vi "Get Signal Names.vi"(8 "error in (no error)":errorcluster, 11 "Incoming/Outgoing in":T1 format="%.0x") -> (0 "error out":errorcluster, 1 "signal names":string[](array[string]), 2 "signals":T1[](array[typedef]) format="%.0x", 3 "Incoming/Outgoing out":T1 format="%.0x")   [LabVIEW 2020, in "Communication Bus Template Engine.lvlib" / "Implementation.lvlib" / "Execution Unit Factory.lvclass"]
uses:
  Execution Unit Factory.lvclass
  Scripting/Communication Bus Template Scripting.lvlib
  <vilib>/NI VeriStand/Custom Device API/Custom Device API.lvlib
  Scripting/Constants.vi
  <vilib>/NI VeriStand/Custom Device Tools/Custom Device Utility Library/Custom Device Utility Library.lvlib
  <vilib>/NI VeriStand/Custom Device Tools/Custom Device Utility Library/NI VeriStand - Search for Item by GUID.vi
  <vilib>/NI VeriStand/Custom Device Tools/Custom Device Utility Library/Search Direction.ctl
  <vilib>/NI VeriStand/Custom Device API/Custom Device Item Ref.ctl
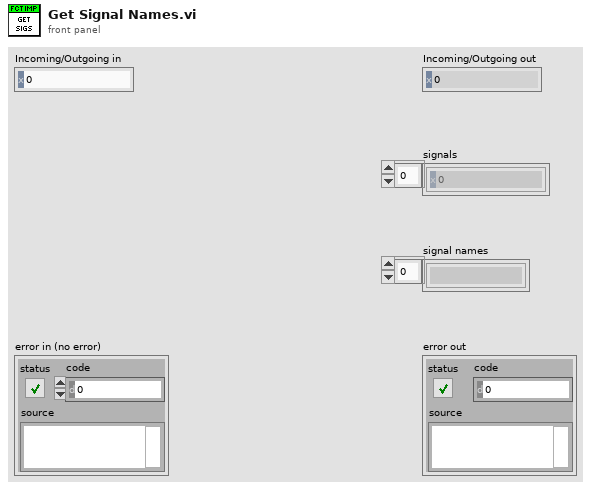
[diagram p1: front panel]
types:
  T1 = typedef "Custom Device API.lvlib/Custom Device Item Ref.ctl" = u64
  T2 = typedef "Custom Device Utility Library.lvlib/Search Direction.ctl" = enum16{"Down", "Up"}
  T3 = typedef "Custom Device API.lvlib/Custom Device Item Info.ctl" = cluster{"Name":string, "Is Channel":bool, "GUID":string, "Is Waveform":bool}
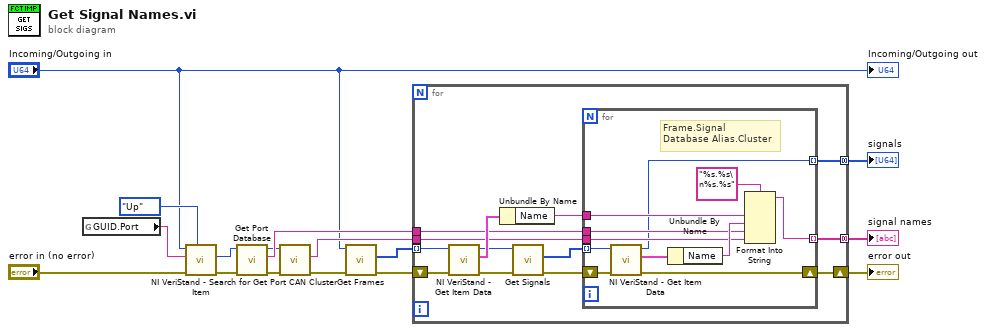
[diagram p0: block diagram]
diagram:
  n1 = global read "Constants.vi" "GUID.Port"() -> (w7:string)
  n2 = call-poly <vilib>:"NI VeriStand - Search for Item.vi"("Direction (Down)"=Search_Direction."Up", "error in"="error in (no error)", "Item GUID"=w7, "Section Ref in"="Incoming/Outgoing in") -> ("error out"=w3:errorcluster, "Item Ref"=w2:T1)  [unwired: 4 in, 2 out]
  n3 = call "Get Port Database.vi"("error in"=w3, "Port Ref"=w2) -> ("error out"=w12:errorcluster, "Database Name"=w15:string, "Port Ref out"=w11:T1)  [unwired: 5 in, 2 out]
  n4 = call "Get Port CAN Cluster.vi"("error in"=w12, "Port Ref"=w11) -> ("error out"=w4:errorcluster, "CAN Cluster"=w16:string)  [unwired: 7 in, 1 out]
  n5 = call "Get Frames.vi"("error in"=w4, "Incoming/Outgoing in"="Incoming/Outgoing in") -> ("error out"=w14:errorcluster, "Frames"=w13:T1[])  [unwired: 7 in, 1 out]
  n6 = for {
    tunnel: w13 -> [w28] mode=indexing
    shift-right: [w26] -> w10
    shift-left: w14 -> [w27]
    tunnel: w15 -> [w17]
    tunnel: w16 -> [w24]
    tunnel: [w23] -> w9 mode=concatenating
    tunnel: [w22] -> w8 mode=concatenating
    n7 = call <vilib>:"NI VeriStand - Get Item Data.vi"("error in (no error)"=w27, "Item Ref in"=w28) -> ("error out"=w20:errorcluster, "Item Info"=w29:T3, "Item Ref out"=w21:T1)  [unwired: 6 in, 1 out]
    n8 = Unbundle By Name(w29) -> ("Name"=w25:string)
    n9 = call "Get Signals.vi"("error in"=w20, "Frame in"=w21) -> ("error out"=w19:errorcluster, "Signals"=w18:T1[])  [unwired: 7 in, 1 out]
    n10 = for {
      shift-right: [w37] -> w26
      shift-left: w19 -> [w38]
      tunnel: w18 -> [w32] mode=indexing
      tunnel: w25 -> [w39]
      tunnel: w17 -> [w34]
      tunnel: w24 -> [w33]
      tunnel: [w31] -> w23 mode=indexing
      tunnel: [w30] -> w22 mode=indexing
      # "Frame.Signal\nDatabase Alias.Cluster"
      n11 = call <vilib>:"NI VeriStand - Get Item Data.vi"("error in (no error)"=w38, "Item Ref in"=w32) -> ("error out"=w37:errorcluster, "Item Info"=w36:T3, "Item Ref out"=w30:T1)  [unwired: 6 in, 1 out]
      n12 = Unbundle By Name(w36) -> ("Name"=w35:string)
      n13 = Format Into String(format string="%s.%s\n%s.%s", w39, w35, w34, w33) -> (resulting string=w31:string)  [unwired: 2 in, 1 out]
    }
  }
  "error out" <- w10
  "signal names" <- w9
  "signals" <- w8
  "Incoming/Outgoing out" <- "Incoming/Outgoing in"
